vi "工位2扫码1.vi"(9 "工位1表格":string[][](array[string]), 11 "MulticolumnListbox输入":refnum<vi>) -> (2 "条码字符串":string, 3 "工位2NG?":bool)   [LabVIEW 2011]
uses:
  <vilib>/Utility/miscctls.llb/LVRowAndColumnTypeDef.ctl
panel:
  in  "多列列表框":i32[](listbox)
  out "条码数组":string[](array[string])
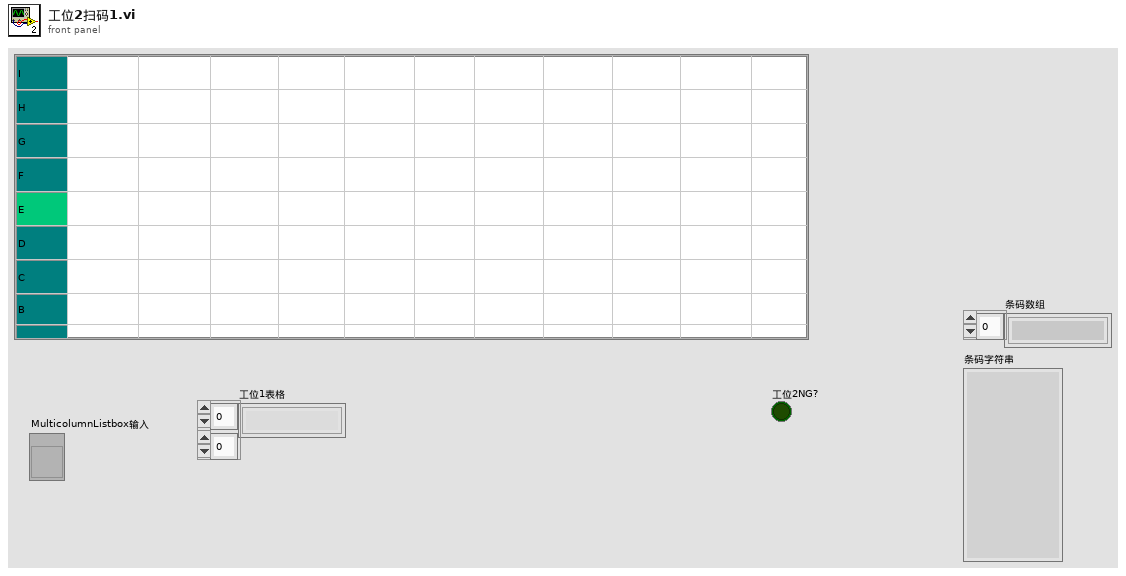
[diagram p1: front panel]
types:
  T1 = typedef "LVRowAndColumnTypeDef.ctl" = cluster{"Row":i32, "Column":i32}
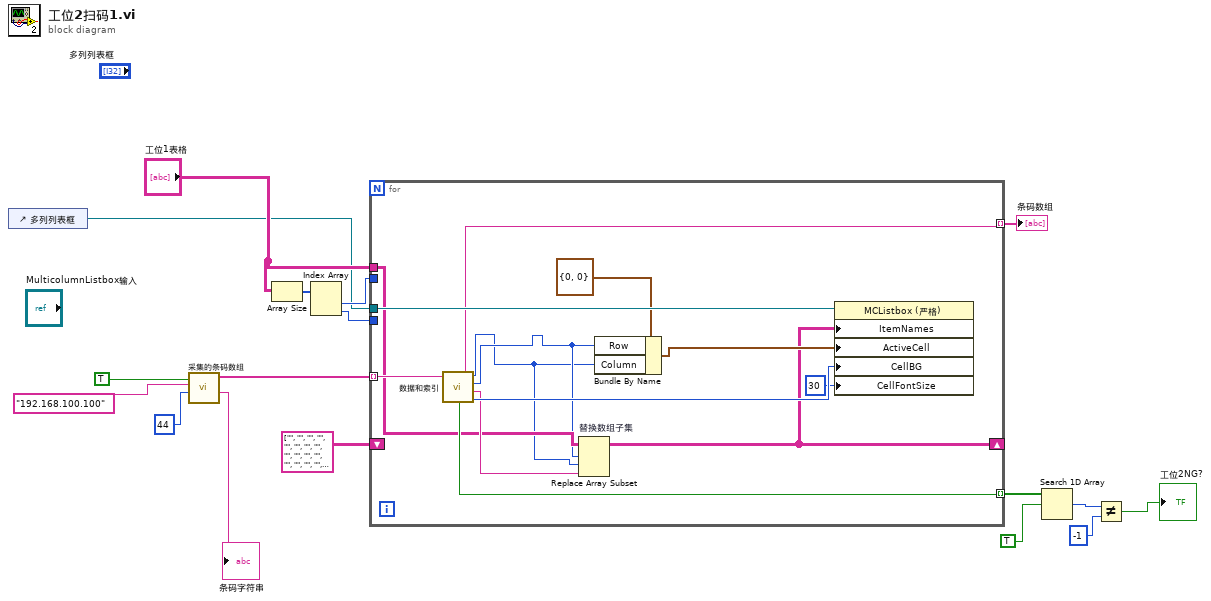
[diagram p0: block diagram]
diagram:
  n1 = control-ref of="多列列表框"() -> (w1:refnum<vi>)
  n2 = call "采集的条码数组.vi"("条码数量"=44, "地址"="192.168.100.100", "开启条码?"=TRUE) -> ("条码字符串"=→"条码字符串":string, "料号"=w15:string[])  [unwired: 6 in, 1 out]
  n3 = Array Size(array="工位1表格") -> (size(s)=w4:i32[])
  n4 = Index Array(array=w4) -> (element #1=w3:i32, element #2=w2:i32)  [unwired: 2 in]
  n5 = for {
    tunnel: w1 -> [w30]
    tunnel: "工位1表格" -> [w21]
    tunnel: w15 -> [w29] mode=indexing
    shift-right: [w22] -> _
    shift-left: string[][] [["", "", "", "", "", "", "", "", "", "", ""], ["", "", "", "", "", "", "", "", "", "", ""], ["", "", "", "", "", "", "", "", "", "", ""], ["", "", "", "", "", "", "", "", "", "", ""], ["", "", "", "", "", "", "", "", "", "", ""]] -> [_]
    tunnel: [w24] -> w13 mode=indexing
    tunnel: [w23] -> w7 mode=indexing
    tunnel: w3 -> [_]
    tunnel: w2 -> [_]
    n6 = call "数据和索引.vi"("data out"=w29) -> ("颜色"=w26:u32, "显示数据"=w25:string, "索引行"=w20:i32, "索引列"=w19:i32, "NG?"=w24:bool, "条码"=w23:string)  [unwired: 5 in]
    n7 = Replace Array Subset "替换数组子集"(array=w21, new element=w25, index (row)=w20, index (col)=w19) -> (w22:string[][])
    n8 = Bundle By Name(cluster=T1 {"Row"=0, "Column"=0} ("活动单元格:活动单元格"), "Row"=w20, "Column"=w19) -> (w28:T1)
    n9 = property class="MCListbox (严格)"(reference=w30, "ItemNames"=w22, "ActiveCell"=w28, "CellBG"=w26, "CellFontSize"=u32 30 ("活动单元格:单元格字体:字号")) -> ()  [unwired: 1 in, 2 out]
  }
  "条码数组" <- w7
  n10 = Search 1D Array(1D array=w13, element=TRUE) -> (index of element=w11:i32)  [unwired: 1 in]
  n11 = Not Equal?(x=w11, y=-1) -> (x != y?=→"工位2NG?":bool)
